vi "Graph Vindu.vi"(1 "Loop ID Master":u16, 2 "Loop ID Slave":u16, 11 "error in (no error)":errorcluster) -> ()   [LabVIEW 2011]
uses:
  Graph/Plot selector.ctl
  <vilib>/picture/picture.llb/imagedata.ctl
  Prod Cons Clust.ctl
  Prod Cons Action.ctl
  Measurments Handling/Action Analog Handler.ctl
  Annotation/Actin Annotatino Holder.ctl
  emi Lib/System 01/0 - General/App/Loop control 2/Private/_emi_SMLoop Control Single.vi
  emi Lib/System 01/0 - General/App/Loop control 2/Private/_emi_ SMLoop start condition.vi
  emi Lib/System 01/0 - General/App/Loop control 2/Private/_emi_ SMLoop Error Check.vi
  emi Lib/Basic/0 - General/Error/emi_Is Error.vi
  emi Lib/System 01/0 - General/App/Loop control 2/Private/_emi_SMLoop Register new.vi
  emi Lib/System 01/0 - General/S&E reporting/emi_Send S&E Error message.vi
  emi Lib/Basic/0 - General/Error/emi_ Is Error state.vi
  emi Lib/System 01/0 - General/emi_Read System ID.vi
  emi Lib/System 01/0 - General/App/Loop control/Private/_emi_GFV Loop Running.vi
  emi Lib/System 01/0 - General/App/Loop control/Private/_emi_GFV Loop Enable.vi
  emi Lib/System 01/0 - General/App/Loop control/Private/_emi_GFV Loop Linking.vi
  emi Lib/System 01/0 - General/App/Loop control 2/Private/_emi_ SMLoop Restart.vi
  emi Lib/System 01/0 - General/App/Loop control/Private/_emi_GFV stop a loop so it can reset.vi
  emi Lib/System 01/0 - General/App/Loop control 2/Private/_emi_ SMLoop Restart Counter.vi
  emi Lib/System 01/0 - General/App/Private/_emi_GFV App Close.vi
  emi Lib/System 01/0 - General/Private/_emi_GFV System ID.vi
  emi Lib/System 01/0 - General/S&E reporting/Private/_emi_S&E Q Generator.vi
panel:
  out "L2":dbl format="%#.2f"
  out "L1":dbl format="%#.2f"
  in  "Plot L2":T1 {"Line Width" items=["0", "1", "2", "3", "4", "5"]; "Var Tag" items=["", "HVPSU Head Voltage(V)", "HVPSU TS Voltage(V)", "HVPSU Current(A)", "PCP Cable Resistance(Ohm)", "Winch Depth(m)", "Winch Line Speed(m/min)", "Winch Wire Tension(kg)", "Tool Max Temperature(degC)", "Tool (Controller) Temperature(degC)", "Tool Supply Voltage(V)", "Tool (Controller) Current(A)", "Tool Acceleration X(g)", "Tool Acceleration Y(g)", "Tool Acceleration Z(g)", "Tool Acceleration Sum(g)", "Tool Inclination(deg)", "Tool Rotation(deg)", "Tool GP Sensor 1(V)", "Tool GP Sensor 2(V)", "Tool (Pressure 1) Temperature(degC)", "Tool Pressure 1 RAW(bar)", "Tool (Pressure 2) Temperature(degC)", "Tool Pressure 2 RAW(bar)", "Tool (Solenoid) Temperature(degC)", "Tool Solenoid Position(m)", "PSU Temp(degC)", "Head Voltage(V)", "PSU Main Voltage out(V)", "PSU Main Current out(A)", "Upper Tension Sub Temp(degC)", "Tool Upper Tension Sub Raw(kg)", "Lower Tension Sub Temp(degC)", "Tool Lower Tension Sub Raw(kg)", "Tool Var27 - Reserved(V)", "Tool Var28 - Reserved(V)", "Tool Var29 - Reserved(V)", "Tool Var30 - Reserved(V)", "Stroke Extension(mm)", "Stroke In Force(tonne)", "Stroke Out Force(tonne)", "Stroke Force(tonne)", "Stroker Pressure 1(bar)", "Stroker Pressure 2(bar)", "Stroker Upper Tension Sub(kg)", "Stroker Lower Tension Sub(kg)", "Stroker Var09 - Reserved(V)", "Stroker Var10 - Reserved(V)", "Tractor Upper Tension Sub(kg)", "Tractor Lower Tension Sub(kg)", "Tractor Var03 - Reserved(V)", "Tractor Var04 - Reserved(V)", "Tool Temperature sensor(degC)", "Tool Motor Voltage(V)", "Tool Motor Current(A)", "Tool Motor Torque(tonne)", "Tool weight on bit(tonne)", "Tool Motor RPM(RPM)", "TS_Signal_Quality(NA)", "TS_PCB_Temp(degC)", "TS_Gain(NA)", "DH_Signal_Quality(NA)", "DH_PCB_Temp(degC)", "DH_Gain(NA)", "Link_Status(NA)"]}
  in  "Plot L1":T1 {"Line Width" items=["0", "1", "2", "3", "4", "5"]; "Var Tag" items=["", "HVPSU Head Voltage(V)", "HVPSU TS Voltage(V)", "HVPSU Current(A)", "PCP Cable Resistance(Ohm)", "Winch Depth(m)", "Winch Line Speed(m/min)", "Winch Wire Tension(kg)", "Tool Max Temperature(degC)", "Tool (Controller) Temperature(degC)", "Tool Supply Voltage(V)", "Tool (Controller) Current(A)", "Tool Acceleration X(g)", "Tool Acceleration Y(g)", "Tool Acceleration Z(g)", "Tool Acceleration Sum(g)", "Tool Inclination(deg)", "Tool Rotation(deg)", "Tool GP Sensor 1(V)", "Tool GP Sensor 2(V)", "Tool (Pressure 1) Temperature(degC)", "Tool Pressure 1 RAW(bar)", "Tool (Pressure 2) Temperature(degC)", "Tool Pressure 2 RAW(bar)", "Tool (Solenoid) Temperature(degC)", "Tool Solenoid Position(m)", "PSU Temp(degC)", "Head Voltage(V)", "PSU Main Voltage out(V)", "PSU Main Current out(A)", "Upper Tension Sub Temp(degC)", "Tool Upper Tension Sub Raw(kg)", "Lower Tension Sub Temp(degC)", "Tool Lower Tension Sub Raw(kg)", "Tool Var27 - Reserved(V)", "Tool Var28 - Reserved(V)", "Tool Var29 - Reserved(V)", "Tool Var30 - Reserved(V)", "Stroke Extension(mm)", "Stroke In Force(tonne)", "Stroke Out Force(tonne)", "Stroke Force(tonne)", "Stroker Pressure 1(bar)", "Stroker Pressure 2(bar)", "Stroker Upper Tension Sub(kg)", "Stroker Lower Tension Sub(kg)", "Stroker Var09 - Reserved(V)", "Stroker Var10 - Reserved(V)", "Tractor Upper Tension Sub(kg)", "Tractor Lower Tension Sub(kg)", "Tractor Var03 - Reserved(V)", "Tractor Var04 - Reserved(V)", "Tool Temperature sensor(degC)", "Tool Motor Voltage(V)", "Tool Motor Current(A)", "Tool Motor Torque(tonne)", "Tool weight on bit(tonne)", "Tool Motor RPM(RPM)", "TS_Signal_Quality(NA)", "TS_PCB_Temp(degC)", "TS_Gain(NA)", "DH_Signal_Quality(NA)", "DH_PCB_Temp(degC)", "DH_Gain(NA)", "Link_Status(NA)"]}
  in  "Refresh Data":bool caption="Inspect Chart"
  out "Cursor time":timestamp format="%<%X %x>T"
  out "R2":dbl format="%#.2f"
  out "R1":dbl format="%#.2f"
  in  "Plot R2":T1 {"Line Width" items=["0", "1", "2", "3", "4", "5"]; "Var Tag" items=["", "HVPSU Head Voltage(V)", "HVPSU TS Voltage(V)", "HVPSU Current(A)", "PCP Cable Resistance(Ohm)", "Winch Depth(m)", "Winch Line Speed(m/min)", "Winch Wire Tension(kg)", "Tool Max Temperature(degC)", "Tool (Controller) Temperature(degC)", "Tool Supply Voltage(V)", "Tool (Controller) Current(A)", "Tool Acceleration X(g)", "Tool Acceleration Y(g)", "Tool Acceleration Z(g)", "Tool Acceleration Sum(g)", "Tool Inclination(deg)", "Tool Rotation(deg)", "Tool GP Sensor 1(V)", "Tool GP Sensor 2(V)", "Tool (Pressure 1) Temperature(degC)", "Tool Pressure 1 RAW(bar)", "Tool (Pressure 2) Temperature(degC)", "Tool Pressure 2 RAW(bar)", "Tool (Solenoid) Temperature(degC)", "Tool Solenoid Position(m)", "PSU Temp(degC)", "Head Voltage(V)", "PSU Main Voltage out(V)", "PSU Main Current out(A)", "Upper Tension Sub Temp(degC)", "Tool Upper Tension Sub Raw(kg)", "Lower Tension Sub Temp(degC)", "Tool Lower Tension Sub Raw(kg)", "Tool Var27 - Reserved(V)", "Tool Var28 - Reserved(V)", "Tool Var29 - Reserved(V)", "Tool Var30 - Reserved(V)", "Stroke Extension(mm)", "Stroke In Force(tonne)", "Stroke Out Force(tonne)", "Stroke Force(tonne)", "Stroker Pressure 1(bar)", "Stroker Pressure 2(bar)", "Stroker Upper Tension Sub(kg)", "Stroker Lower Tension Sub(kg)", "Stroker Var09 - Reserved(V)", "Stroker Var10 - Reserved(V)", "Tractor Upper Tension Sub(kg)", "Tractor Lower Tension Sub(kg)", "Tractor Var03 - Reserved(V)", "Tractor Var04 - Reserved(V)", "Tool Temperature sensor(degC)", "Tool Motor Voltage(V)", "Tool Motor Current(A)", "Tool Motor Torque(tonne)", "Tool weight on bit(tonne)", "Tool Motor RPM(RPM)", "TS_Signal_Quality(NA)", "TS_PCB_Temp(degC)", "TS_Gain(NA)", "DH_Signal_Quality(NA)", "DH_PCB_Temp(degC)", "DH_Gain(NA)", "Link_Status(NA)"]}
  in  "Plot  R1":T1 {"Line Width" items=["0", "1", "2", "3", "4", "5"]; "Var Tag" items=["", "HVPSU Head Voltage(V)", "HVPSU TS Voltage(V)", "HVPSU Current(A)", "PCP Cable Resistance(Ohm)", "Winch Depth(m)", "Winch Line Speed(m/min)", "Winch Wire Tension(kg)", "Tool Max Temperature(degC)", "Tool (Controller) Temperature(degC)", "Tool Supply Voltage(V)", "Tool (Controller) Current(A)", "Tool Acceleration X(g)", "Tool Acceleration Y(g)", "Tool Acceleration Z(g)", "Tool Acceleration Sum(g)", "Tool Inclination(deg)", "Tool Rotation(deg)", "Tool GP Sensor 1(V)", "Tool GP Sensor 2(V)", "Tool (Pressure 1) Temperature(degC)", "Tool Pressure 1 RAW(bar)", "Tool (Pressure 2) Temperature(degC)", "Tool Pressure 2 RAW(bar)", "Tool (Solenoid) Temperature(degC)", "Tool Solenoid Position(m)", "PSU Temp(degC)", "Head Voltage(V)", "PSU Main Voltage out(V)", "PSU Main Current out(A)", "Upper Tension Sub Temp(degC)", "Tool Upper Tension Sub Raw(kg)", "Lower Tension Sub Temp(degC)", "Tool Lower Tension Sub Raw(kg)", "Tool Var27 - Reserved(V)", "Tool Var28 - Reserved(V)", "Tool Var29 - Reserved(V)", "Tool Var30 - Reserved(V)", "Stroke Extension(mm)", "Stroke In Force(tonne)", "Stroke Out Force(tonne)", "Stroke Force(tonne)", "Stroker Pressure 1(bar)", "Stroker Pressure 2(bar)", "Stroker Upper Tension Sub(kg)", "Stroker Lower Tension Sub(kg)", "Stroker Var09 - Reserved(V)", "Stroker Var10 - Reserved(V)", "Tractor Upper Tension Sub(kg)", "Tractor Lower Tension Sub(kg)", "Tractor Var03 - Reserved(V)", "Tractor Var04 - Reserved(V)", "Tool Temperature sensor(degC)", "Tool Motor Voltage(V)", "Tool Motor Current(A)", "Tool Motor Torque(tonne)", "Tool weight on bit(tonne)", "Tool Motor RPM(RPM)", "TS_Signal_Quality(NA)", "TS_PCB_Temp(degC)", "TS_Gain(NA)", "DH_Signal_Quality(NA)", "DH_PCB_Temp(degC)", "DH_Gain(NA)", "Link_Status(NA)"]}
  out "Graph 1":waveform(sgl)[](graph)
  in  "Anotations":i32[](listbox)
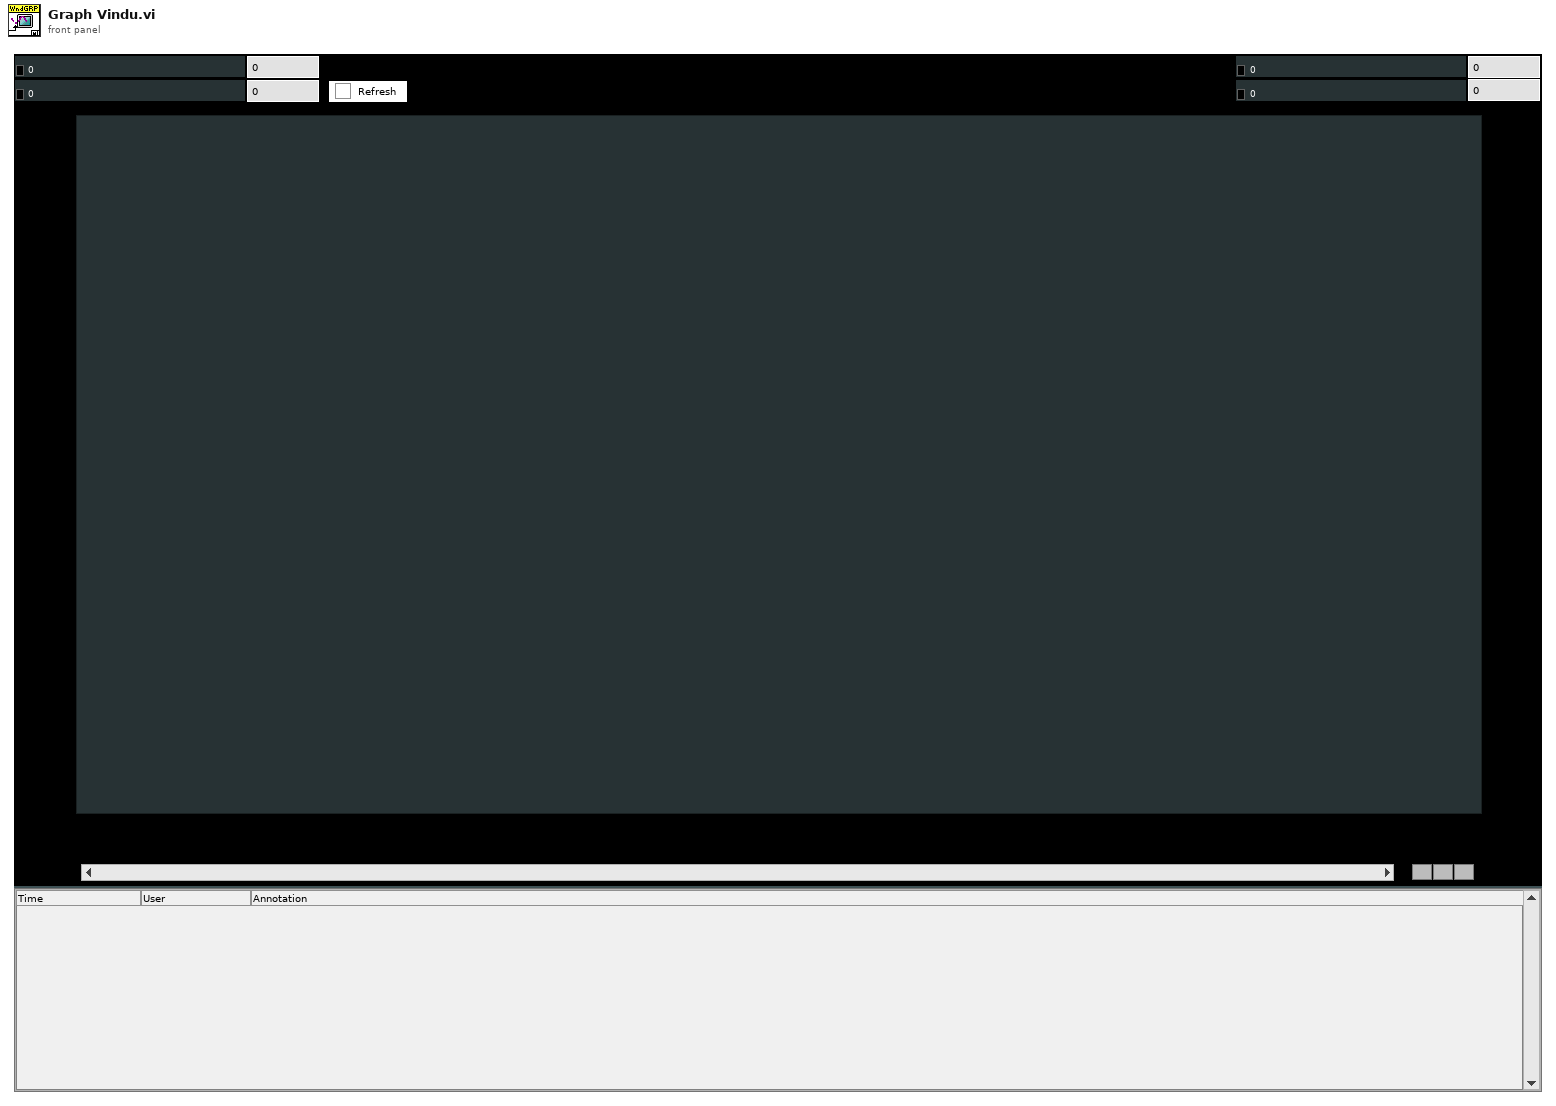
[diagram p1: front panel]
types:
  T1 = typedef "Plot selector.ctl" = cluster{"Var Tag":u16, "Color":u32, "Line Width":u16}
  T2 = typedef "imagedata.ctl" = cluster{"image type":i32, "image depth":i32, "image":u8[], "mask":u8[], "colors":u32[], "Rectangle":cluster{"left":i16, "top":i16, "right":i16, "bottom":i16}}
  T3 = typedef "Action Analog Handler.ctl" = enum16{"GET value", "GET Single Frequenzy", "GET All Values", "GET Waveform", "Get Numb Var", "SET Value", "START Buffer", "REG Variable", "BUF size(total antal sekund)", "PULS", "Get a Value at time", "Set initial waveform"}
  T4 = enum32{"Invalid", "Default", "Floating", "Floating/Auto-Hide", "Modal"}
  T5 = typedef "Prod Cons Action.ctl" = enum16{"Update Graph Data", "Clear Graph", "Setup Graph", "Show Window", "Hide Window", "Load Dropdown lister", "Get Data at Cursor time", "Move Cursor to visible", "Fill anotation list", "Set list values", "Set Graph X-Scale", "Set Graph Y-Scale"}
  T6 = typedef "Prod Cons Clust.ctl" = cluster{"Action":T5, "Data":variant}
  T7 = typedef "Actin Annotatino Holder.ctl" = enum16{"GET Single", "GET All", "GET Time Period", "GET Index", "Get Size", "Add Single", "Replace Single", "Delete Single", "SET All"}
  T8 = enum8{"Enabled", "Disabled", "Disabled and Grayed Out"}
  T9 = enum16{"GET", "SET", "Get from Ini", "Put in Ini"}
  T10 = typedef "_emi_ SMLoop sates.ctl" = enum16{"Init", "Standby", "Start", "Normal Operation", "Stop", "Error Handling", "End", "Post"}
  T11 = typedef "User Setting Analog Channel Bg.ctl" = cluster{"Scaling":T12, "Limits and responces":T13, "Allow Graph selection by user":bool, "Unit":u16}
  T12 = typedef "Scaling.ctl" = cluster{"Gain":dbl, "Offset":dbl}
  T13 = typedef "Alarm Setup Analog.ctl" = cluster{"Technical Error(NA)":T14, "LL":T14, "L":T14, "H":T14, "HH":T14, "Limits":T16}
  T14 = typedef "Alarm Responce.ctl" = cluster{"Action":T15, "Alarm":bool}
  T15 = typedef "Action List.ctl" = enum16{"No Action", "Stop Motor", "Turn Off HV"}
  T16 = typedef "Limits.ctl" = cluster{"LL":dbl, "L":dbl, "H":dbl, "HH":dbl}
  T17 = typedef "Settigner fra Main.ctl" = cluster{"Start Time":timestamp, "Numb Sec Shown":i32, "Plot  L1":T1, "Plot  L2":T1, "Plot  R1":T1, "Plot  R2":T1, "Left Y-scale":T18, "Right Y-scale":T18}
  T18 = typedef "Y scale cluster.ctl" = cluster{"Maximum":dbl, "Minimum":dbl, "Autoscaling":i32}
  T19 = typedef "Annotation Message.ctl" = cluster{"Annotation":string, "User":string, "time":timestamp}
  T20 = typedef "User Indikator.ctl" = cluster{"User Name":string, "Super User":T21}
  T21 = typedef "Super User bool indikator.ctl" = bool
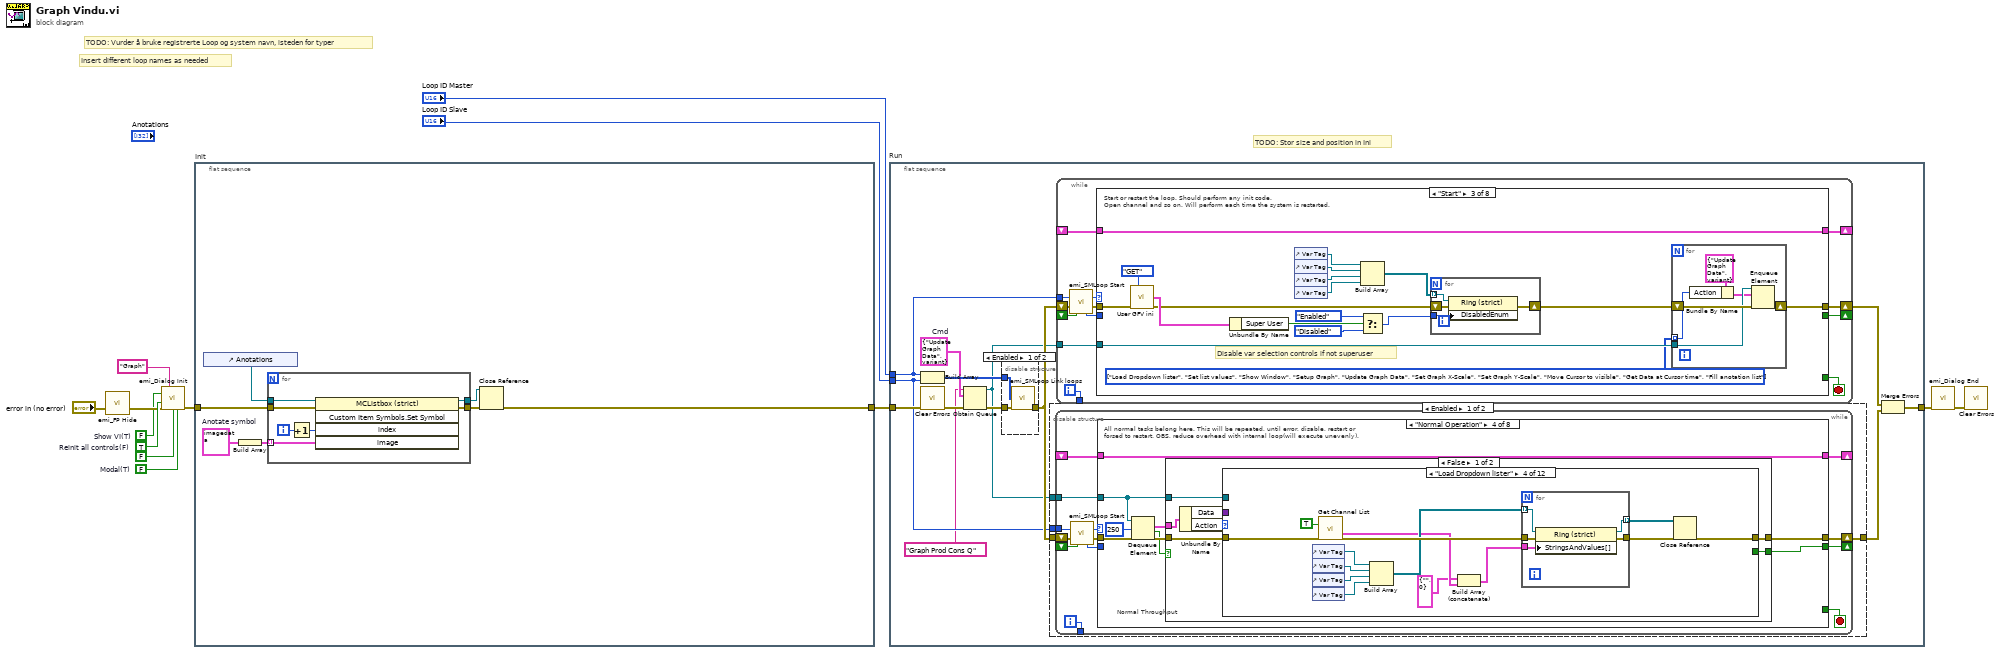
[diagram p0: block diagram]
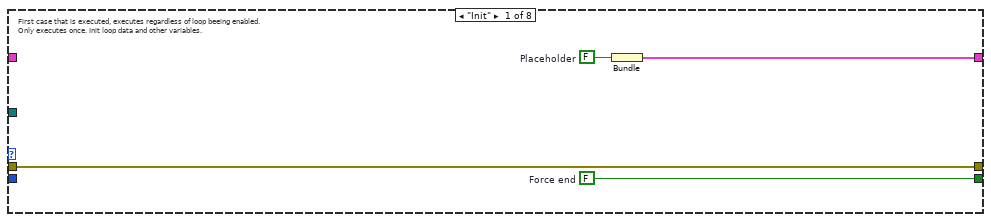
[diagram p2: hidden frame]
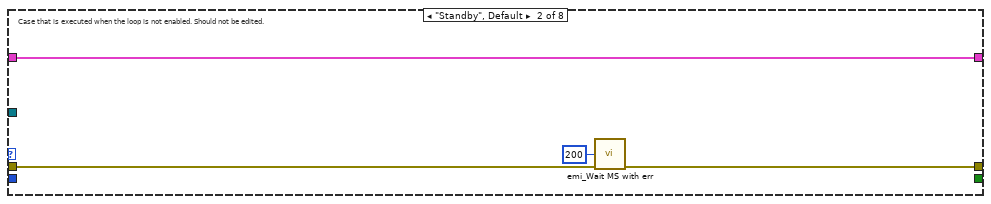
[diagram p3: hidden frame]
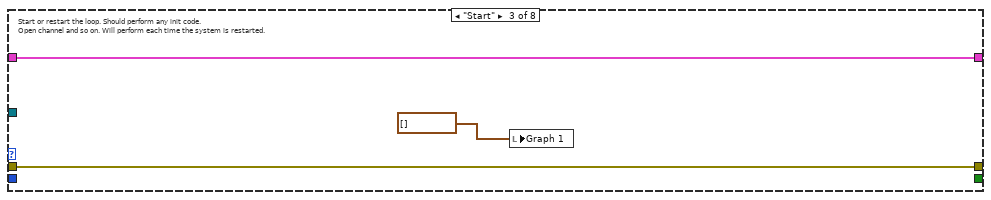
[diagram p4: hidden frame]
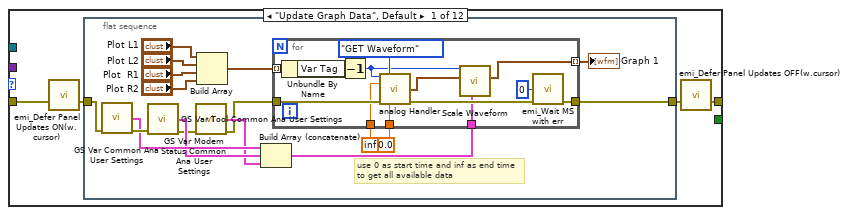
[diagram p5: hidden frame]
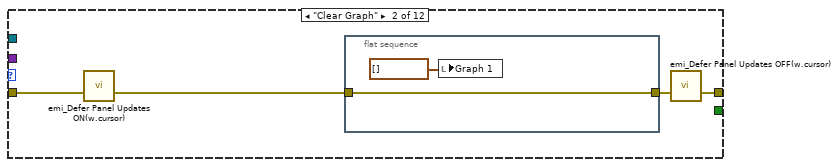
[diagram p6: hidden frame]
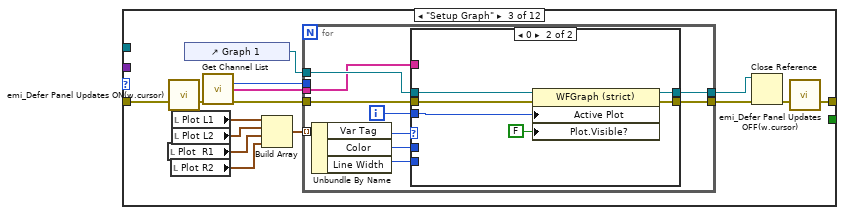
[diagram p7: hidden frame]
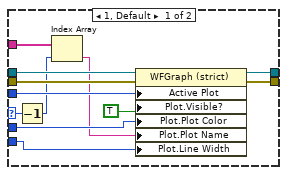
[diagram p8: hidden frame]
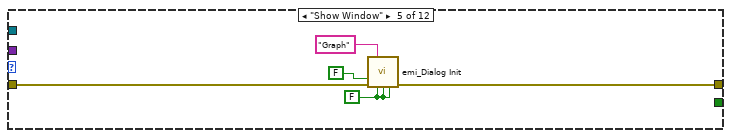
[diagram p9: hidden frame]
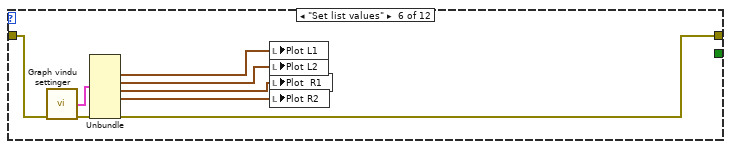
[diagram p10: hidden frame]
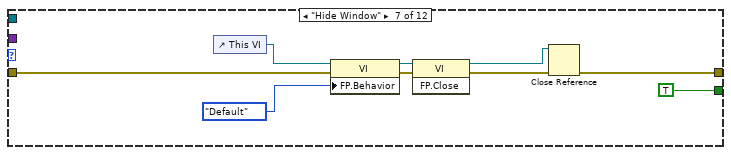
[diagram p11: hidden frame]
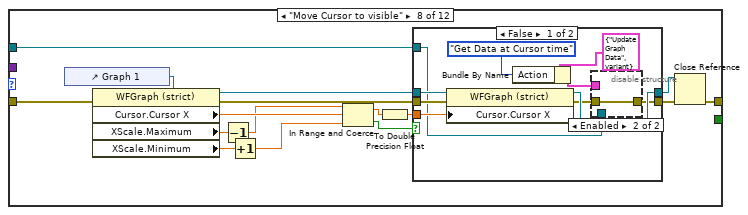
[diagram p12: hidden frame]
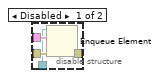
[diagram p13: hidden frame]
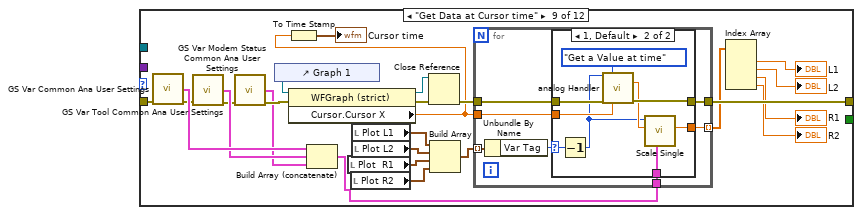
[diagram p15: hidden frame]
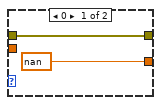
[diagram p16: hidden frame]
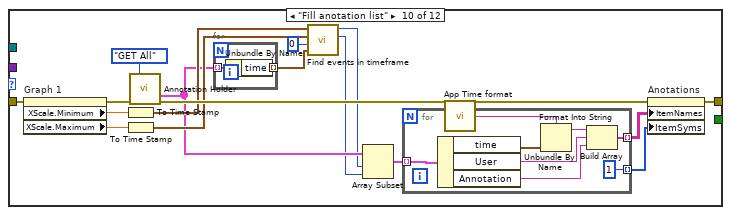
[diagram p17: hidden frame]
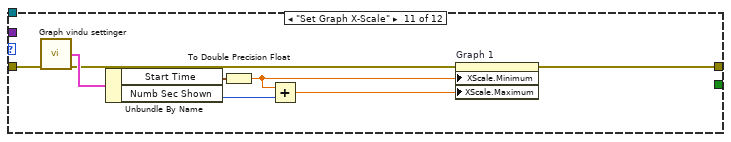
[diagram p18: hidden frame]
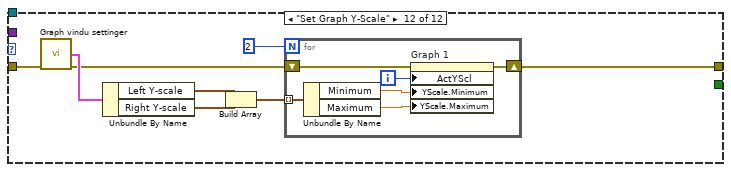
[diagram p19: hidden frame]
diagram:
  w8 = FALSE  # Show VI(T)
  w11 = TRUE  # Reinit all controls(F)
  w12 = FALSE  # Modal(T)
  # "TODO: Stor size and position in Ini"
  # "TODO: Vurder å bruke registrerte Loop og system navn, isteden for typer"
  # "Insert different loop names as needed"
  n1 = call "emi_FP Hide.vi"("error in (no error)"="error in (no error)") -> ("error out"=w10:errorcluster)  [unwired: 13 in, 1 out]
  n2 = call "emi_Dialog Init.vi"("Header String(\"\")"="Graph" ("Header String(\"\")"), "Show VI(T)"=w8, "Reinit all controls(F)"=w11, "error in"=w10, "Set BG Color(T)"=FALSE, "Modal(T)"=w12) -> ("error out"=w9:errorcluster)  [unwired: 9 in]
  n3 = flat-sequence "Init" {
    tunnel: [w14] -> w4
    tunnel: w9 -> [w18]
    frame #0 {
      w20 = T2 {"image type"=0, "image depth"=32, "image"=[0, 0, 0, 0, 0, 0, 0, 0, 0, 0, 0, 0, 255, 47, 45, 155, 255, 0, 0, 128, 255, 0, 0, 128, 255, 0, 0, 128, 255, 47, 45, 155, 255, 204, 199, 240, 0, 0, 0, 0, 0, 0, 0, 0, 0, 0, 0, 0, 0, 0, 0, 0, 0, 0, 0, 0, 0, 0, 0, 0, 0, 0, 0, 0, 0, 0, 0, 0, 255, 95, 92, 183, 255, 87, 77, 183, 255, 255, 255, 255, 255, 255, 255, 255, 255, 255, 255, 255, 255, 255, 255, 255, 255, 255, 255, 255, 255, 87, 77, 183, 255, 95, 93, 183, 0, 0, 0, 0, 0, 0, 0, 0, 0, 0, 0, 0, 0, 0, 0, 0, 0, 0, 0, 0, 0, 0, 0, 0, 255, 98, 93, 184, 255, 255, 255, 255, 255, 255, 255, 255, 255, 255, 255, 255, 255, 255, 255, 255, 255, 255, 255, 255, 255, 255, 255, 255, 255, 255, 255, 255, 255, 255, 255, 255, 255, 255, 255, 255, 255, 98, 93, 184, 0, 0, 0, 0, 0, 0, 0, 0, 0, 0, 0, 0, 0, 0, 0, 0, 0, 0, 0, 0, 255, 35, 29, 154, 255, 255, 255, 255, 255, 255, 255, 255, 255, 255, 255, 255, 255, 255, 255, 255, 255, 255, 255, 255, 255, 255, 255, 255, 255, 255, 255, 255, 255, 255, 255, 255, 255, 255, 255, 255, 255, 72, 58, 181, 0, 0, 0, 0, 0, 0, 0, 0, 0, 0, 0, 0, 0, 0, 0, 0, 0, 0, 0, 0, 255, 30, 28, 155, 255, 255, 254, 245, 255, 255, 255, 255, 255, 255, 255, 255, 255, 255, 255, 255, 255, 255, 255, 255, 255, 255, 255, 255, 255, 255, 255, 255, 255, 255, 255, 255, 255, 255, 254, 245, 255, 61, 57, 178, 0, 0, 0, 0, 0, 0, 0, 0, 0, 0, 0, 0, 0, 0, 0, 0, 0, 0, 0, 0, 0, 0, 0, 0, 255, 76, 75, 182, 255, 114, 105, 184, 255, 255, 255, 255, 255, 255, 255, 255, 255, 255, 255, 255, 255, 255, 255, 255, 255, 255, 255, 255, 255, 114, 105, 184, 255, 77, 75, 177, 0, 0, 0, 0, 0, 0, 0, 0, 0, 0, 0, 0, 0, 0, 0, 0, 0, 0, 0, 0, 0, 0, 0, 0, 0, 0, 0, 0, 0, 0, 0, 0, 0, 0, 0, 0, 255, 70, 68, 180, 255, 255, 254, 254, 255, 255, 255, 255, 255, 244, 229, 255, 255, 67, 68, 180, 0, 0, 0, 0, 0, 0, 0, 0, 0, 0, 0, 0, 0, 0, 0, 0, 0, 0, 0, 0, 0, 0, 0, 0, 0, 0, 0, 0, 0, 0, 0, 0, 0, 0, 0, 0, 0, 0, 0, 0, 0, 0, 0, 0, 0, 0, 0, 0, 255, 83, 81, 180, 255, 255, 255, 255, 255, 83, 75, 177, 0, 0, 0, 0, 0, 0, 0, 0, 255, 204, 164, 58, 255, 255, 210, 87, 255, 255, 215, 108, 255, 255, 207, 78, 255, 204, 182, 124, 0, 0, 0, 0, 0, 0, 0, 0, 0, 0, 0, 0, 0, 0, 0, 0, 0, 0, 0, 0, 0, 0, 0, 0, 0, 0, 0, 0, 255, 91, 81, 182, 255, 33, 25, 149, 0, 0, 0, 0, 255, 204, 182, 124, 255, 255, 236, 186, 255, 255, 238, 193, 255, 255, 223, 135, 255, 255, 206, 73, 255, 255, 196, 36, 255, 204, 182, 124, 0, 0, 0, 0, 0, 0, 0, 0, 0, 0, 0, 0, 0, 0, 0, 0, 0, 0, 0, 0, 0, 0, 0, 0, 0, 0, 0, 0, 255, 89, 88, 173, 255, 90, 89, 168, 255, 255, 215, 108, 255, 255, 241, 203, 255, 255, 238, 191, 255, 255, 222, 135, 255, 255, 206, 72, 255, 255, 189, 9, 255, 203, 167, 68, 0, 0, 0, 0, 0, 0, 0, 0, 0, 0, 0, 0, 0, 0, 0, 0, 0, 0, 0, 0, 0, 0, 0, 0, 0, 0, 0, 0, 0, 0, 0, 0, 0, 0, 0, 0, 255, 255, 210, 89, 255, 255, 227, 151, 255, 255, 225, 145, 255, 255, 215, 105, 255, 255, 201, 52, 255, 255, 187, 1, 255, 255, 212, 97, 0, 0, 0, 0, 0, 0, 0, 0, 0, 0, 0, 0, 0, 0, 0, 0, 0, 0, 0, 0, 0, 0, 0, 0, 0, 0, 0, 0, 0, 0, 0, 0, 0, 0, 0, 0, 255, 229, 182, 53, 255, 255, 208, 82, 255, 255, 208, 78, 255, 255, 200, 50, 255, 255, 190, 13, 255, 255, 187, 4, 255, 229, 193, 95, 0, 0, 0, 0, 0, 0, 0, 0, 0, 0, 0, 0, 0, 0, 0, 0, 0, 0, 0, 0, 0, 0, 0, 0, 0, 0, 0, 0, 0, 0, 0, 0, 0, 0, 0, 0, 0, 0, 0, 0, 255, 234, 187, 42, 255, 255, 193, 22, 255, 255, 189, 9, 255, 255, 187, 1, 255, 230, 181, 26, 0, 0, 0, 0, 0, 0, 0, 0, 0, 0, 0, 0, 0, 0, 0, 0, 0, 0, 0, 0, 0, 0, 0, 0, 0, 0, 0, 0, 0, 0, 0, 0, 0, 0, 0, 0, 0, 0, 0, 0, 255, 63, 116, 153, 255, 121, 141, 94, 255, 210, 170, 29, 255, 217, 173, 25, 255, 195, 165, 38, 255, 85, 126, 110, 255, 33, 94, 132, 0, 0, 0, 0, 0, 0, 0, 0, 0, 0, 0, 0, 0, 0, 0, 0, 0, 0, 0, 0, 0, 0, 0, 0, 0, 0, 0, 0, 0, 0, 0, 0, 255, 161, 196, 221, 255, 161, 196, 221, 255, 113, 166, 204, 255, 70, 139, 188, 255, 42, 121, 178, 255, 23, 109, 171, 255, 8, 101, 166, 255, 2, 97, 164, 255, 100, 158, 199, 0, 0, 0, 0, 0, 0, 0, 0, 0, 0, 0, 0, 0, 0, 0, 0, 0, 0, 0, 0, 0, 0, 0, 0, 0, 0, 0, 0, 255, 161, 196, 221, 255, 161, 196, 221, 255, 113, 166, 204, 255, 70, 139, 188, 255, 42, 121, 178, 255, 23, 109, 171, 255, 8, 101, 166, 255, 2, 97, 164, 255, 61, 134, 185], "mask"=[31, 128, 127, 192, 255, 224, 255, 224, 255, 224, 127, 192, 31, 0, 14, 124, 6, 254, 3, 254, 0, 254, 0, 254, 0, 124, 0, 254, 1, 255, 1, 255], "colors"=[], "Rectangle"={"left"=0, "top"=0, "right"=16, "bottom"=16}}  # Anotate symbol
      n4 = control-ref of="Anotations"() -> (w16:refnum<vi>)
      n5 = Build Array(w20) -> (w19:T2[])
      n6 = for {
        tunnel: w16 -> [w27]
        tunnel: w19 -> [w24] mode=indexing
        tunnel: w18 -> [w23]
        tunnel: [w22] -> w17
        tunnel: [w21] -> w15
        i -> [w26]
        n7 = Increment(x=w26) -> (x+1=w25:i32)
        n8 = invoke class="MCListbox (strict)" method="Custom Item Symbols.Set Symbol"(reference=w27, error in=w23, "index"=w25, "image"=w24) -> (reference out=w21:refnum<vi>, error out=w22:errorcluster)  [unwired: 1 in, 3 out]
      }
      n9 = Close Reference(reference=w15, error in (no error)=w17) -> (error out=w14:errorcluster)
    }
  }
  n10 = flat-sequence "Run" {
    tunnel: w4 -> [w40]
    tunnel: [w37] -> w7
    tunnel: "Loop ID Master" -> [w35]
    tunnel: "Loop ID Slave" -> [w34]
    frame #0 {
      w30 = T6 {"Action"=enum."Update Graph Data", "Data"=variant}  # Cmd
      n11 = Build Array(w35, w34) -> (w33:u16[])
      n12 = call <vilib>:"Clear Errors.vi"("error in (no error)"=w40) -> ("error out"=w31:errorcluster)  [unwired: 6 in]
      n13 = Obtain Queue(name (unnamed)="Graph Prod Cons Q", element data type=w30, error in (no error)=w31) -> (queue out=w28:refnum<queue>, error out=w32:errorcluster)  [unwired: 2 in, 1 out]
      n14 = disable-structure shown="Enabled" {
        disable-tunnel: w32 -> [w347 w348]
        disable-tunnel: [w346 w348] -> w36
        disable-tunnel: w33 -> [w345 _]
        frame Enabled {
          n15 = call "emi_SMLoop Link loops.vi"("Loop IDS"=w345, "error in (no error)"=w347) -> ("error out"=w346:errorcluster)  [unwired: 13 in]
        }
        frame Disabled {
        }
      }
      n16 = disable-structure shown="Enabled" {
        disable-tunnel: [w44 w344] -> w38
        disable-tunnel: w36 -> [w43 w344]
        disable-tunnel: w34 -> [w42 _]
        disable-tunnel: w28 -> [w41 _]
        frame Enabled {
          n17 = while {
            shift-right: [w57] -> _
            shift-left: _ -> [w53]
            shift-right: [w55] -> w44
            shift-left: w43 -> [w51]
            tunnel: [w54] -> _
            shift-right: [w52] -> _
            shift-left: _ -> [w47]
            tunnel: w42 -> [w48]
            tunnel: w41 -> [w45]
            i -> [w54]
            stop <- w56 stop-if-true
            n18 = call "emi_SMLoop Start.vi"("Loop ID"=w48, "error in (no error)"=w51, "Force Stop(F)"=w47) -> ("Loop command"=w49:T10, "error out"=w50:errorcluster, "Loop ID out"=w46:i32)  [unwired: 10 in]
            n19 = case shown="\"Normal Operation\"" w49 {
              tunnel: [w61 w62 w68 w75 w335 w338 w339 w342] -> w57
              tunnel: [_ _ _ _ _ _ _ TRUE] -> w56
              tunnel: w50 -> [w58 w64 w67 w77 w336 w337 w340 w343]
              tunnel: [w58 w63 w67 w76 w336 w337 w340 w343] -> w55
              tunnel: w53 -> [_ w62 w68 w75 w335 w338 w339 w342]
              tunnel: [w59 _ _ w74 _ _ _ _] -> w52
              tunnel: w46 -> [_ _ _ _ _ _ _ _]
              tunnel: w45 -> [_ _ _ w73 _ _ _ _]
              frame "Init" {
                w59 = FALSE  # Force end
                w60 = FALSE  # Placeholder
                # "First case that is executed, executes regardless of loop beeing enabled.\nOnly executes once. Init loop data and other variables."
                n20 = Bundle("Placeholder"=w60) -> (w61:cluster{"Placeholder":bool})  [unwired: 1 in]
              }
              frame "Standby", Default {
                # "Case that is executed when the loop is not enabled. Should not be edited."
                n21 = call "emi_Wait MS with err.vi"("milliseconds to wait(0)"=u32 200, "error in (no error)"=w64) -> ("error out"=w63:errorcluster)  [unwired: 13 in]
              }
              frame "Start" {
                # "Start or restart the loop. Should perform any init code. \nOpen channel and so on. Will perform each time the system is restarted."
                n22 = local write "Graph 1"(waveform(sgl)[] [] ("Chart 1")) -> ()
              }
              frame "Normal Operation" {
                # "Normal Throughput"
                # "All normal tasks belong here. This will be repeated, until error, disable, restart or\nforsed to restart. OBS, reduce overhead with internal loop(will execute unevenly)."
                n23 = Dequeue Element(queue=w73, timeout in ms (-1)=250, error in (no error)=w77) -> (element=w69:T6, timed out?=w70:bool, error out=w71:errorcluster)  [unwired: 1 out]
                n24 = case shown="False" w70 {
                  tunnel: w71 -> [w84 w333]
                  tunnel: [w83 w333] -> w76
                  tunnel: w69 -> [w82 _]
                  tunnel: [w79 _] -> w74
                  tunnel: w73 -> [w78 _]
                  frame False {
                    n25 = Unbundle By Name(w82) -> ("Data"=w80:variant, "Action"=w81:T5)
                    n26 = case shown="\"Load Dropdown lister\"" w81 {
                      tunnel: w84 -> [w88 w122 w139 w177 w190 w198 w204 w223 w246 w285 w318 w326]
                      tunnel: [w85 w119 w138 w176 w189 w197 w202 w221 w257 w286 w311 w323] -> w83
                      tunnel: w80 -> [_ _ _ _ _ _ _ _ _ _ _ _]
                      tunnel: [_ _ _ _ _ _ TRUE ("Force End") _ _ _ _ _] -> w79
                      tunnel: w78 -> [_ _ _ _ _ _ _ w213 _ _ _ _]
                      frame "Update Graph Data", Default {
                        n27 = call "emi_Defer Panel Updates ON(w.cursor).vi"("error in (no error)"=w88) -> ("error out"=w87:errorcluster)  [unwired: 13 in, 1 out]
                        n28 = flat-sequence {
                          tunnel: w87 -> [w95]
                          tunnel: [w105] -> w86
                          frame #0 {
                            # "use 0 as start time and inf as end time\nto get all available data"
                            n29 = call "GS Var Common Ana User Settings.vi"("error in (no error)"=w95) -> ("Common Analog var User set out"=w97:T11[], "error out"=w98:errorcluster)  [unwired: 12 in, 1 out]
                            n30 = call "GS Var Tool Common Ana User Settings.vi"("error in (no error)"=w98) -> ("Tool Analog var User settigns out"=w96:T11[], "error out"=w91:errorcluster)  [unwired: 12 in, 1 out]
                            n31 = call "GS Var Modem Status Common Ana User Settings.vi"("error in (no error)"=w91) -> ("Modem Status Analog var User settigns out"=w90:T11[], "error out"=w89:errorcluster)  [unwired: 12 in, 1 out]
                            n32 = Build Array("Plot L1", "Plot L2", "Plot  R1", "Plot R2") -> (w104:T1[])
                            n33 = Build Array (concatenate)(w97, w96, w90) -> (w94:T11[])
                            n34 = for {
                              tunnel: w89 -> [w118]
                              tunnel: [w113] -> w105
                              tunnel: 0.0 -> [w111]
                              tunnel: inf -> [w116]
                              tunnel: w104 -> [w115] mode=indexing
                              tunnel: [w109] -> w103 mode=indexing
                              tunnel: w94 -> [w107]
                              n35 = Unbundle By Name(w115) -> ("Var Tag"=w108:u16)
                              n36 = Decrement(x=w108) -> (x-1=w106:u16)
                              n37 = call "analog Handler.vi"("Variable Index"=w106, "Action"=Action_Analog_Handler."GET Waveform" ("Action(GET)"), "End Tid"=w116, "error in (no error)"=w118, "Start tid / buf size"=w111) -> ("Waveform"=w110:waveform(sgl), "error out"=w117:errorcluster)  [unwired: 5 in, 4 out]
                              n38 = call "Scale Waveform.vi"("Variable Configuration"=w107, "Waveform"=w110, "Var Tag"=w106) -> ("output waveform"=w109:waveform(sgl))  [unwired: 8 in]
                              n39 = call "emi_Wait MS with err.vi"("milliseconds to wait(0)"=u32 0, "error in (no error)"=w117) -> ("error out"=w113:errorcluster)  [unwired: 13 in]
                            }
                            "Graph 1" <- w103
                          }
                        }
                        n40 = call "emi_Defer Panel Updates OFF(w.cursor).vi"("error in (no error)"=w86) -> ("error out"=w85:errorcluster)  [unwired: 13 in, 1 out]
                      }
                      frame "Clear Graph" {
                        n41 = call "emi_Defer Panel Updates ON(w.cursor).vi"("error in (no error)"=w122) -> ("error out"=w121:errorcluster)  [unwired: 13 in, 1 out]
                        n42 = flat-sequence {
                          tunnel: w121 -> [w123]
                          tunnel: [w123] -> w120
                          frame #0 {
                            n43 = local write "Graph 1"(waveform(sgl)[] [] ("Graph 1")) -> ()
                          }
                        }
                        n44 = call "emi_Defer Panel Updates OFF(w.cursor).vi"("error in (no error)"=w120) -> ("error out"=w119:errorcluster)  [unwired: 13 in, 1 out]
                      }
                      frame "Setup Graph" {
                        n45 = local read "Plot  R1"() -> (w134:T1)
                        n46 = call "emi_Defer Panel Updates ON(w.cursor).vi"("error in (no error)"=w139) -> ("error out"=w137:errorcluster)  [unwired: 13 in, 1 out]
                        n47 = local read "Plot R2"() -> (w133:T1)
                        n48 = local read "Plot L1"() -> (w136:T1)
                        n49 = local read "Plot L2"() -> (w135:T1)
                        n50 = control-ref of="Graph 1"() -> (w126:refnum<vi>)
                        n51 = call "Get Channel List.vi"("error in"=w137) -> ("Numb Elements"=w129:i32, "Names"=w130:string[], "error out"=w132:errorcluster)  [unwired: 10 in, 2 out]
                        n52 = Build Array(w136, w135, w134, w133) -> (w131:T1[])
                        n53 = for {
                          tunnel: w132 -> [w149]
                          tunnel: w131 -> [w144] mode=indexing
                          tunnel: w130 -> [w141]
                          tunnel: w129 -> [_]
                          tunnel: [w148] -> w127
                          tunnel: w126 -> [w147]
                          tunnel: [w146] -> w125
                          i -> [w145]
                          n54 = Unbundle By Name(w144) -> ("Var Tag"=w142:u16, "Color"=w143:u32, "Line Width"=w140:u16)
                          n55 = case shown="0" w142 {
                            selector: w142 -> [w153 _]
                            tunnel: w149 -> [w161 w167]
                            tunnel: [w160 w166] -> w148
                            tunnel: w147 -> [w159 w165]
                            tunnel: [w158 w164] -> w146
                            tunnel: w145 -> [w157 w163]
                            tunnel: w143 -> [w155 _]
                            tunnel: w141 -> [w154 _]
                            tunnel: w140 -> [w150 _]
                            frame 1, Default {
                              n56 = Decrement(x=w153) -> (x-1=w152:u16)
                              n57 = Index Array(array=w154, index=w152) -> (element=w151:string)
                              n58 = property class="WFGraph (strict)"(reference=w159, error in=w161, "Active Plot"=w157, "Plot.Visible?"=TRUE ("Plot.Visible"), "Plot.Plot Color"=w155, "Plot.Plot Name"=w151, "Plot.Line Width"=w150) -> (reference out=w158:refnum<vi>, error out=w160:errorcluster)
                            }
                            frame 0 {
                              n59 = property class="WFGraph (strict)"(reference=w165, error in=w167, "Active Plot"=w163, "Plot.Visible?"=FALSE ("Plot.Visible")) -> (reference out=w164:refnum<vi>, error out=w166:errorcluster)
                            }
                          }
                        }
                        n60 = Close Reference(reference=w125, error in (no error)=w127) -> (error out=w128:errorcluster)
                        n61 = call "emi_Defer Panel Updates OFF(w.cursor).vi"("error in (no error)"=w128) -> ("error out"=w138:errorcluster)  [unwired: 13 in, 1 out]
                      }
                      frame "Load Dropdown lister" {
                        n62 = control-ref of="Var Tag"() -> (w175:refnum<vi>)
                        n63 = control-ref of="Var Tag"() -> (w174:refnum<vi>)
                        n64 = control-ref of="Var Tag"() -> (w173:refnum<vi>)
                        n65 = control-ref of="Var Tag"() -> (w172:refnum<vi>)
                        n66 = call "Get Channel List.vi"("Force all(F)"=TRUE, "error in"=w177) -> ("Ring list"=w170:cluster{"String":string, "Value":u16}[], "error out"=w181:errorcluster)  [unwired: 9 in, 3 out]
                        n67 = Build Array(w175, w174, w173, w172) -> (w171:refnum<vi>[])
                        n68 = Build Array (concatenate)(cluster{"String":string, "Value":i32} {"String"="", "Value"=0}, w170) -> (w178:cluster{"String":string, "Value":i32}[])
                        n69 = for {
                          tunnel: w181 -> [w186]
                          tunnel: w178 -> [w182]
                          tunnel: w171 -> [w183] mode=indexing
                          tunnel: [w185] -> w180
                          tunnel: [w184] -> w179 mode=indexing
                          n70 = property class="Ring (strict)"(reference=w183, error in=w186, "StringsAndValues[]"=w182) -> (reference out=w184:refnum<vi>, error out=w185:errorcluster)
                        }
                        n71 = Close Reference(reference=w179, error in (no error)=w180) -> (error out=w176:errorcluster)
                      }
                      frame "Show Window" {
                        w187 = FALSE ("Set BG Color(T)")
                        n72 = call "emi_Dialog Init.vi"("Header String(\"\")"="Graph" ("Header String(\"\")"), "Reinit all controls(F)"=FALSE, "error in"=w190, "Center in bottom FP(T)"=w187, "Set BG Color(T)"=w187, "Modal(T)"=w187) -> ("error out"=w189:errorcluster)  [unwired: 9 in]
                      }
                      frame "Set list values" {
                        n73 = call "Graph vindu settinger.vi"("error in (no error)"=w198) -> ("Settigner fra MAin out"=w196:T17, "error out"=w197:errorcluster)  [unwired: 13 in]
                        n74 = Unbundle(w196) -> ("Plot  L1"=w195:T1, "Plot  L2"=w194:T1, "Plot  R1"=w193:T1, "Plot  R2"=w192:T1)  [unwired: 4 out]
                        n75 = local write "Plot L1"(w195) -> ()
                        n76 = local write "Plot L2"(w194) -> ()
                        n77 = local write "Plot  R1"(w193) -> ()
                        n78 = local write "Plot R2"(w192) -> ()
                      }
                      frame "Hide Window" {
                        n79 = control-ref of="This VI"() -> (w201:refnum<vi>)
                        n80 = property class="VI"(reference=w201, error in=w204, "FP.Behavior"=T4."Default" ("Front Panel Window:Behavior")) -> (reference out=w205:refnum<vi>, error out=w206:errorcluster)
                        n81 = invoke class="VI" method="FP.Close"(reference=w205, error in=w206) -> (reference out=w199:refnum<vi>, error out=w203:errorcluster)  [unwired: 1 in, 1 out]
                        n82 = Close Reference(reference=w199, error in (no error)=w203) -> (error out=w202:errorcluster)
                      }
                      frame "Move Cursor to visible" {
                        n83 = control-ref of="Graph 1"() -> (w222:refnum<vi>)
                        n84 = property class="WFGraph (strict)"(reference=w222, error in=w223) -> (reference out=w219:refnum<vi>, error out=w220:errorcluster, "Cursor.Cursor X"=w212:dbl, "XScale.Maximum"=w211:dbl, "XScale.Minimum"=w210:dbl)
                        n85 = Decrement(x=w211) -> (x-1=w208:dbl)
                        n86 = Increment(x=w210) -> (x+1=w209:dbl)
                        n87 = In Range and Coerce(upper limit=w208, x=w212, lower limit=w209) -> (coerced(x)=w216:dbl, In Range?=w214:bool)
                        n88 = To Double Precision Float(number=w216) -> (double precision float=w215:dbl)
                        n89 = case shown="False" w214 {
                          tunnel: w220 -> [w233 w239]
                          tunnel: w219 -> [w232 w240]
                          tunnel: [w230 w240] -> w218
                          tunnel: [w227 w239] -> w217
                          tunnel: w215 -> [w231 _]
                          tunnel: w213 -> [w225 _]
                          frame False {
                            n90 = property class="WFGraph (strict)"(reference=w232, error in=w233, "Cursor.Cursor X"=w231) -> (reference out=w230:refnum<vi>, error out=w228:errorcluster)
                            n91 = Bundle By Name(cluster=T6 {"Action"=enum."Update Graph Data", "Data"=variant} ("element"), "Action"=Prod_Cons_Action."Get Data at Cursor time") -> (w229:T6)
                            n92 = disable-structure shown="Enabled" {
                              disable-tunnel: w229 -> [w237 _]
                              disable-tunnel: w228 -> [w236 w238]
                              disable-tunnel: [w235 w238] -> w227
                              disable-tunnel: w225 -> [w234 _]
                              frame Disabled {
                                n93 = Enqueue Element(queue=w234, element=w237, error in (no error)=w236) -> (error out=w235:errorcluster)  [unwired: 1 in, 2 out]
                              }
                              frame Enabled {
                              }
                            }
                          }
                          frame True {
                          }
                        }
                        n94 = Close Reference(reference=w218, error in (no error)=w217) -> (error out=w221:errorcluster)
                      }
                      frame "Get Data at Cursor time" {
                        n95 = call "GS Var Common Ana User Settings.vi"("error in (no error)"=w246) -> ("Common Analog var User set out"=w248:T11[], "error out"=w245:errorcluster)  [unwired: 12 in, 1 out]
                        n96 = call "GS Var Tool Common Ana User Settings.vi"("error in (no error)"=w245) -> ("Tool Analog var User settigns out"=w247:T11[], "error out"=w243:errorcluster)  [unwired: 12 in, 1 out]
                        n97 = call "GS Var Modem Status Common Ana User Settings.vi"("error in (no error)"=w243) -> ("Modem Status Analog var User settigns out"=w241:T11[], "error out"=w242:errorcluster)  [unwired: 12 in, 1 out]
                        n98 = control-ref of="Graph 1"() -> (w265:refnum<vi>)
                        n99 = property class="WFGraph (strict)"(reference=w265, error in=w242) -> (reference out=w263:refnum<vi>, error out=w264:errorcluster, "Cursor.Cursor X"=w250:dbl)
                        n100 = To Time Stamp(1:w250) -> (0:→"Cursor time":timestamp)
                        n101 = Build Array (concatenate)(w248, w247, w241) -> (w244:T11[])
                        n102 = local read "Plot  R1"() -> (w261:T1)
                        n103 = local read "Plot R2"() -> (w262:T1)
                        n104 = local read "Plot L1"() -> (w259:T1)
                        n105 = local read "Plot L2"() -> (w260:T1)
                        n106 = Close Reference(reference=w263, error in (no error)=w264) -> (error out=w256:errorcluster)
                        n107 = Build Array(w259, w260, w261, w262) -> (w258:T1[])
                        n108 = for {
                          tunnel: w258 -> [w272] mode=indexing
                          tunnel: [w269] -> w257
                          tunnel: w256 -> [w270]
                          tunnel: w250 -> [w268]
                          tunnel: [w267] -> w255 mode=indexing
                          tunnel: w244 -> [w266]
                          n109 = Unbundle By Name(w272) -> ("Var Tag"=w271:u16)
                          n110 = case shown="1, Default" w271 {
                            selector: w271 -> [_ w283]
                            tunnel: w270 -> [w274 w282]
                            tunnel: [w274 w281] -> w269
                            tunnel: [nan w277] -> w267
                            tunnel: w268 -> [_ w279]
                            tunnel: w266 -> [_ w275]
                            frame 0 {
                            }
                            frame 1, Default {
                              n111 = Decrement(x=w283) -> (x-1=w276:u16)
                              n112 = call "analog Handler.vi"("Variable Index"=w276, "Action"=Action_Analog_Handler."Get a Value at time", "error in (no error)"=w282, "Start tid / buf size"=w279) -> ("Value out"=w278:dbl, "error out"=w281:errorcluster)  [unwired: 6 in, 4 out]
                              n113 = call "Scale Single.vi"("Variable Configuration"=w275, "Unscaled data in"=w278, "Var Tag"=w276) -> ("Scaled data out"=w277:dbl)  [unwired: 8 in]
                            }
                          }
                        }
                        n114 = Index Array(array=w255) -> (element #1=→"L1":dbl, element #2=→"L2":dbl, element #3=→"R1":dbl, element #4=→"R2":dbl)  [unwired: 4 in]
                      }
                      frame "Fill anotation list" {
                        n115 = property on="Graph 1" class="WFGraph (strict)"(error in=w285) -> (error out=w284:errorcluster, "XScale.Minimum"=w296:dbl, "XScale.Maximum"=w295:dbl)  [unwired: 1 in, 1 out]
                        n116 = To Time Stamp(1:w296) -> (0:w294:timestamp)
                        n117 = To Time Stamp(1:w295) -> (0:w293:timestamp)
                        n118 = call "Annotation Holder.vi"("Action"=Actin_Annotatino_Holder."GET All", "error in (no error)"=w284) -> ("Array Of annotations"=w290:T19[], "error out"=w299:errorcluster)  [unwired: 9 in, 3 out]
                        n119 = for {
                          tunnel: w290 -> [w302] mode=indexing
                          tunnel: [w301] -> w291 mode=indexing
                          n120 = Unbundle By Name(w302) -> ("time"=w301:timestamp)
                        }
                        n121 = call "Find events in timeframe.vi"("Data Array"=w291, "Offset in"=0, "End time"=w293, "Start time"=w294) -> ("length out"=w288:i32, "index out"=w289:i32)  [unwired: 5 in, 1 out]
                        n122 = Array Subset(array=w290, index=w289, length=w288) -> (w287:T19[])
                        n123 = for {
                          tunnel: w287 -> [w308] mode=indexing
                          tunnel: [1] -> w298 mode=indexing
                          tunnel: [w309] -> w297 mode=indexing
                          n124 = Unbundle By Name(w308) -> ("time"=w303:timestamp, "User"=w306:string, "Annotation"=w307:string)
                          n125 = call "App Time format.vi"() -> ("App timeformat"=w304:string)  [unwired: 15 in]
                          n126 = Format Into String(format string=w304, w303) -> (resulting string=w305:string)  [unwired: 2 in, 1 out]
                          n127 = Build Array(w305, w306, w307) -> (w309:string[])
                        }
                        n128 = property on="Anotations" class="MCListbox (strict)"(error in=w299, "ItemNames"=w297, "ItemSyms"=w298) -> (error out=w286:errorcluster)  [unwired: 1 in, 1 out]
                      }
                      frame "Set Graph X-Scale" {
                        n129 = call "Graph vindu settinger.vi"("error in (no error)"=w318) -> ("Settigner fra MAin out"=w317:T17, "error out"=w312:errorcluster)  [unwired: 13 in]
                        n130 = Unbundle By Name(w317) -> ("Start Time"=w315:timestamp, "Numb Sec Shown"=w316:i32)
                        n131 = To Double Precision Float(number=w315) -> (double precision float=w313:dbl)
                        n132 = Add(x=w313, y=w316) -> (x+y=w314:dbl)
                        n133 = property on="Graph 1" class="WFGraph (strict)"(error in=w312, "XScale.Minimum"=w313, "XScale.Maximum"=w314) -> (error out=w311:errorcluster)  [unwired: 1 in, 1 out]
                      }
                      frame "Set Graph Y-Scale" {
                        n134 = call "Graph vindu settinger.vi"("error in (no error)"=w326) -> ("Settigner fra MAin out"=w325:T17, "error out"=w324:errorcluster)  [unwired: 13 in]
                        n135 = Unbundle By Name(w325) -> ("Left Y-scale"=w321:T18, "Right Y-scale"=w320:T18)
                        n136 = Build Array(w321, w320) -> (w319:T18[])
                        n137 = for {
                          N: 2 -> [_]
                          shift-right: [w331] -> w323
                          shift-left: w324 -> [w332]
                          tunnel: w319 -> [w329] mode=indexing
                          i -> [w330]
                          n138 = Unbundle By Name(w329) -> ("Minimum"=w328:dbl, "Maximum"=w327:dbl)
                          n139 = property on="Graph 1" class="WFGraph (strict)"(error in=w332, "ActYScl"=w330, "YScale.Minimum"=w328, "YScale.Maximum"=w327) -> (error out=w331:errorcluster)  [unwired: 1 in, 1 out]
                        }
                      }
                    }
                  }
                  frame True {
                    # "Timeout"
                  }
                }
              }
              frame "Stop" {
                # "To alow VI to exit befor \nAplicatin End.\nFor use in dialogs"
                # "Stop the loop. May be restarted later. Close interfaces and the like"
                n140 = local write "Graph 1"(waveform(sgl)[] [] ("Chart 1")) -> ()
              }
              frame "Error Handling" {
                # "Loop automaticaly returns here after error is found. If error is cleared, \nLoop wil continue as normal(if was operative when error."
              }
              frame "End" {
                # "Only executes at application end has. Should performa any action the loop \nneeds to finnish. Executes only once."
              }
              frame "Post" {
                # "Only exists to pas true to loop conditional without extra VI. DO Not edit"
              }
            }
          }
        }
        frame Disabled {
        }
      }
      n141 = while {
        shift-right: [w361] -> _
        shift-left: _ -> [w357]
        shift-right: [w359] -> w39
        shift-left: w36 -> [w355]
        tunnel: [w358] -> _
        shift-right: [w356] -> _
        shift-left: _ -> [w351]
        tunnel: w35 -> [w352]
        tunnel: w28 -> [w349]
        i -> [w358]
        stop <- w360 stop-if-true
        n142 = call "emi_SMLoop Start.vi"("Loop ID"=w352, "error in (no error)"=w355, "Force Stop(F)"=w351) -> ("Loop command"=w353:T10, "error out"=w354:errorcluster, "Loop ID out"=w350:i32)  [unwired: 10 in]
        n143 = case shown="\"Start\"" w353 {
          tunnel: [w364 w366 w387 w402 w482 w484 w485 w488] -> w361
          tunnel: [_ _ _ _ _ _ _ TRUE] -> w360
          tunnel: w354 -> [w365 w368 w382 w404 w481 w483 w486 w489]
          tunnel: [w365 w367 w385 w403 w478 w483 w486 w489] -> w359
          tunnel: w357 -> [_ w366 w387 w401 w482 w484 w485 w488]
          tunnel: [w362 _ _ w400 _ _ _ _] -> w356
          tunnel: w350 -> [_ _ _ _ w480 _ _ _]
          tunnel: w349 -> [_ _ w386 w399 _ _ _ _]
          frame "Init" {
            w362 = FALSE  # Force end
            w363 = FALSE  # Delayed update
            # "First case that is executed, executes regardless of loop beeing enabled.\nOnly executes once. Init loop data and other variables."
            n144 = Bundle("Delayed update"=w363) -> (w364:cluster{"Delayed update":bool})  [unwired: 1 in]
          }
          frame "Standby", Default {
            # "Case that is executed when the loop is not enabled. Should not be edited."
            n145 = call "emi_Wait MS with err.vi"("milliseconds to wait(0)"=u32 200, "error in (no error)"=w368) -> ("error out"=w367:errorcluster)  [unwired: 13 in]
          }
          frame "Start" {
            w384 = T5[] [enum."Load Dropdown lister", enum."Set list values", enum."Show Window", enum."Setup Graph", enum."Update Graph Data", enum."Set Graph X-Scale", enum."Set Graph Y-Scale", enum."Move Cursor to visible", enum."Get Data at Cursor time", enum."Fill anotation list"] items=["Update Graph Data", "Clear Graph", "Setup Graph", "Show Window", "Hide Window", "Load Dropdown lister", "Get Data at Cursor time", "Move Cursor to visible", "Fill anotation list", "Set list values", "Set Graph X-Scale", "Set Graph Y-Scale"]
            # "Disable var selection controls if not superuser"
            # "Start or restart the loop. Should perform any init code. \nOpen channel and so on. Will perform each time the system is restarted."
            n146 = call "User GFV ini.vi"("Action(GET)"=T9."GET", "error in (no error)"=w382) -> ("User ID out"=w381:T20, "error out"=w380:errorcluster)  [unwired: 12 in]
            n147 = Unbundle By Name(w381) -> ("Super User"=w377:T21)
            n148 = control-ref of="Var Tag"() -> (w373:refnum<vi>)
            n149 = control-ref of="Var Tag"() -> (w372:refnum<vi>)
            n150 = control-ref of="Var Tag"() -> (w371:refnum<vi>)
            n151 = control-ref of="Var Tag"() -> (w370:refnum<vi>)
            n152 = Build Array(w373, w372, w371, w370) -> (w378:refnum<vi>[])
            n153 = Select(t=T8."Enabled" ("Disabled"), s=w377, f=T8."Disabled" ("Disabled")) -> (s? t:f=w374:T8)
            n154 = for {
              tunnel: w378 -> [w391] mode=indexing
              tunnel: w374 -> [w390]
              shift-right: [w389] -> w379
              shift-left: w380 -> [w388]
              n155 = property class="Ring (strict)"(reference=w391, error in=w388, "DisabledEnum"=w390) -> (error out=w389:errorcluster)  [unwired: 1 out]
            }
            n156 = for {
              tunnel: w386 -> [w396]
              tunnel: w384 -> [w393] mode=indexing
              shift-right: [w392] -> w385
              shift-left: w379 -> [w397]
              n157 = Bundle By Name(cluster=T6 {"Action"=enum."Update Graph Data", "Data"=variant} ("element"), "Action"=w393) -> (w394:T6)
              n158 = Enqueue Element(queue=w396, element=w394, error in (no error)=w397) -> (error out=w392:errorcluster)  [unwired: 1 in, 2 out]
            }
          }
          frame "Normal Operation" {
            # "All normal tasks belong here. This will be repeated, until error, disable, restart or\nforsed to restart. OBS, reduce overhead with internal loop(will execute unevenly)."
            n159 = event shown="[0] Timeout" {
              selector: _ -> [_ _ _ _ _ _]
              dyn-events: _ -> [_ _ _ _ _ _]
              timeout: 100 -> [_ _ _ _ _ _]
              tunnel: w404 -> [w405 w430 w439 w455 w464 w474]
              tunnel: w401 -> [w410 w434 w444 w457 w467 w476]
              tunnel: [w408 w434 w444 w457 w466 w476] -> w402
              tunnel: [w407 w427 w435 w454 w464 w473] -> w403
              tunnel: [_ FALSE ("Discard?") _ _ _ _] -> w400
              tunnel: w399 -> [w406 w426 w438 w453 _ w471]
              event Timeout {
                n160 = event-data() -> ()  [unwired: 1 in, 1 out]
                n161 = Unbundle By Name(w410) -> ("Delayed update"=w409:bool)
                n162 = case shown="True" w409 {
                  tunnel: w410 -> [w412 w419]
                  tunnel: [w412 w418] -> w408
                  tunnel: [w411 w416] -> w407
                  tunnel: w406 -> [_ w415]
                  tunnel: w405 -> [w411 w414]
                  frame False {
                  }
                  frame True {
                    w413 = T5[] [enum."Move Cursor to visible", enum."Get Data at Cursor time", enum."Fill anotation list"] items=["Update Graph Data", "Clear Graph", "Setup Graph", "Show Window", "Hide Window", "Load Dropdown lister", "Get Data at Cursor time", "Move Cursor to visible", "Fill anotation list", "Set list values", "Set Graph X-Scale", "Set Graph Y-Scale"]
                    n163 = for {
                      tunnel: w415 -> [w424]
                      shift-right: [w425] -> w416
                      shift-left: w414 -> [w423]
                      tunnel: w413 -> [w420] mode=indexing
                      n164 = Bundle By Name(cluster=T6 {"Action"=enum."Update Graph Data", "Data"=variant} ("element"), "Action"=w420) -> (w421:T6)
                      n165 = Enqueue Element(queue=w424, element=w421, error in (no error)=w423) -> (error out=w425:errorcluster)  [unwired: 1 in, 2 out]
                    }
                    n166 = Bundle By Name(cluster=w419, "Delayed update"=FALSE) -> (w418:cluster{"Delayed update":bool})
                  }
                }
              }
              event Panel Close? {
                n167 = event-data() -> ()  [unwired: 1 in, 1 out]
                n168 = Bundle By Name(cluster=T6 {"Action"=enum."Update Graph Data", "Data"=variant} ("element"), "Action"=Prod_Cons_Action."Hide Window") -> (w431:T6)
                n169 = Enqueue Element(queue=w426, element=w431, error in (no error)=w430) -> (error out=w427:errorcluster)  [unwired: 1 in, 2 out]
                n170 = event-data("Discard?"=TRUE) -> ()  [unwired: 1 in, 1 out]
              }
              event Value Change {
                n171 = event-data() -> ("OldVal"=w442:T1, "NewVal"=w443:T1)  [unwired: 1 in]
                n172 = Unbundle By Name(w442) -> ("Var Tag"=w440:u16)
                n173 = Unbundle By Name(w443) -> ("Var Tag"=w441:u16)
                n174 = Not Equal?(x=w440, y=w441) -> (x != y?=w437:bool)
                n175 = case shown="True" w437 {
                  tunnel: [w445 w446] -> w436
                  frame False {
                    w445 = T5[] [enum."Setup Graph"] items=["Update Graph Data", "Clear Graph", "Setup Graph", "Show Window", "Hide Window", "Load Dropdown lister", "Get Data at Cursor time", "Move Cursor to visible", "Fill anotation list", "Set list values", "Set Graph X-Scale", "Set Graph Y-Scale"]
                  }
                  frame True {
                    w446 = T5[] [enum."Clear Graph", enum."Setup Graph", enum."Update Graph Data", enum."Move Cursor to visible", enum."Get Data at Cursor time"] items=["Update Graph Data", "Clear Graph", "Setup Graph", "Show Window", "Hide Window", "Load Dropdown lister", "Get Data at Cursor time", "Move Cursor to visible", "Fill anotation list", "Set list values", "Set Graph X-Scale", "Set Graph Y-Scale"]
                  }
                }
                n176 = for {
                  tunnel: w439 -> [w452]
                  tunnel: w438 -> [w451]
                  tunnel: w436 -> [w448] mode=indexing
                  tunnel: [w447] -> w435
                  n177 = Bundle By Name(cluster=T6 {"Action"=enum."Update Graph Data", "Data"=variant} ("element"), "Action"=w448) -> (w449:T6)
                  n178 = Enqueue Element(queue=w451, element=w449, error in (no error)=w452) -> (error out=w447:errorcluster)  [unwired: 1 in, 2 out]
                }
              }
              event "Refresh Data": Value Change {
                w456 = T5[] [enum."Update Graph Data"] items=["Update Graph Data", "Clear Graph", "Setup Graph", "Show Window", "Hide Window", "Load Dropdown lister", "Get Data at Cursor time", "Move Cursor to visible", "Fill anotation list", "Set list values", "Set Graph X-Scale", "Set Graph Y-Scale"]
                # "Loads the most recent data into the graph, but does not change the time axis"
                n179 = event-data() -> ()  [unwired: 1 in, 1 out]
                n180 = for {
                  tunnel: w455 -> [w463]
                  tunnel: w453 -> [w462]
                  tunnel: w456 -> [w459] mode=indexing
                  tunnel: [w458] -> w454
                  n181 = Bundle By Name(cluster=T6 {"Action"=enum."Update Graph Data", "Data"=variant} ("element"), "Action"=w459) -> (w460:T6)
                  n182 = Enqueue Element(queue=w462, element=w460, error in (no error)=w463) -> (error out=w458:errorcluster)  [unwired: 1 in, 2 out]
                }
              }
              event "Graph 1": Scale Range Change {
                # "Some of the Range Change origins can fire off multiple events rapidly. It is not worth updating all properties for each event."
                n183 = event-data() -> ()  [unwired: 1 in, 1 out]
                n184 = Bundle By Name(cluster=w467, "Delayed update"=TRUE) -> (w466:cluster{"Delayed update":bool})
              }
              event "Graph 1": Cursor Move; "Graph 1": Cursor Release {
                n185 = event-data() -> ()  [unwired: 1 in, 1 out]
                n186 = Bundle By Name(cluster=T6 {"Action"=enum."Update Graph Data", "Data"=variant} ("element"), "Action"=Prod_Cons_Action."Get Data at Cursor time") -> (w468:T6)
                n187 = Enqueue Element(queue=w471, element=w468, error in (no error)=w474) -> (error out=w475:errorcluster)  [unwired: 1 in, 2 out]
                n188 = call "emi_Wait MS with err.vi"("milliseconds to wait(0)"=u32 1, "error in (no error)"=w475) -> ("error out"=w473:errorcluster)  [unwired: 13 in]
              }
            }
          }
          frame "Stop" {
            # "Så ikke auto starter igjen om enablet"
            # "To alow VI to exit befor \nAplicatin End.\nFor use in dialogs"
            # "Stop the loop. May be restarted later. Close interfaces and the like"
            n189 = call-poly "emi_SMLoop Control.vi"("Loop ID in"=w480, "Enable"=FALSE, "error in (no error)"=w481) -> ("error out"=w479:errorcluster)  [unwired: 11 in, 1 out]
            n190 = call "emi_FP Hide.vi"("error in (no error)"=w479) -> ("error out"=w478:errorcluster)  [unwired: 13 in, 1 out]
          }
          frame "Error Handling" {
            # "Loop automaticaly returns here after error is found. If error is cleared, \nLoop wil continue as normal(if was operative when error."
          }
          frame "End" {
            # "Only executes at application end has. Should performa any action the loop \nneeds to finnish. Executes only once."
          }
          frame "Post" {
            # "Only exists to pas true to loop conditional without extra VI. DO Not edit"
          }
        }
      }
      n191 = Merge Errors(w39, w38) -> (w37:errorcluster)
    }
  }
  n192 = call "emi_Dialog End.vi"("error in"=w7) -> ("error out"=w3:errorcluster)  [unwired: 14 in]
  n193 = call <vilib>:"Clear Errors.vi"("error in (no error)"=w3) -> ()  [unwired: 6 in, 1 out]
